vi "check chassis status.vi"(8 "error in (no error)":errorcluster {"code" format="%.0x"}, 11 "resource name":string="PXI11::0::0::INSTR" caption="resource string") -> (0 "error out":errorcluster {"code" format="%.0x"}, 3 "Status OK":bool)   [LabVIEW 2023]
uses:
  Program Files (x86)/Keysight/MPxiChassis/LabVIEW Driver/20xx/Keysight MPxiChassis/Keysight MPxiChassis.lvlib
panel:
  out "AlarmOccurred":bool caption="ClockAlarmOccurred"
  out "Clock source":i32=2
  # "0 10MHz from chassis\n1 10MHz clock from external\n2 10MHz from timing module\n3 10MHz clock from high performance reference\n4 2.4GHz clock from high performance reference"
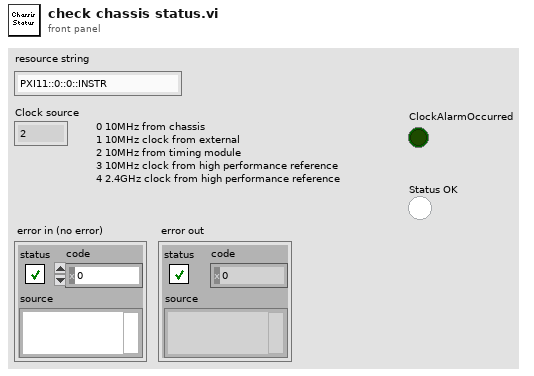
[diagram p1: front panel]
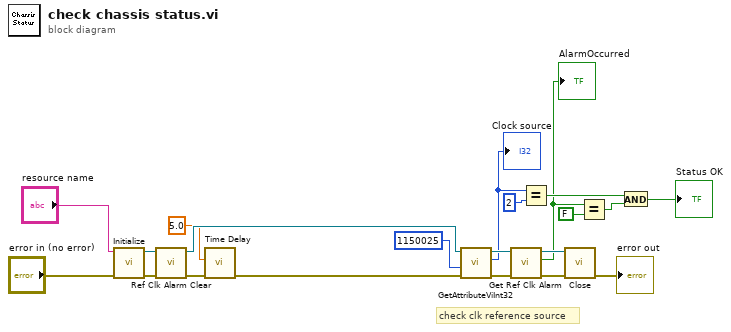
[diagram p0: block diagram]
diagram:
  # "check clk reference source"
  n1 = call "Initialize.vi"("error in (no error)"="error in (no error)", "resource name"="resource name") -> ("error out"=w4:errorcluster, "instrument handle out"=w6:refnum<k15>)  [unwired: 8 in]
  n2 = call "Ref Clk Alarm Clear.vi"("error in (no error)"=w4, "instrument handle"=w6) -> ("error out"=w2:errorcluster, "instrument handle out"=w5:refnum<k15>)  [unwired: 8 in]
  n3 = call "Time Delay"("error in (no error)"=w2, "Delay Time (s)"=5.0) -> ("error out"=w1:errorcluster)  [unwired: 9 in]
  n4 = call "GetAttributeViInt32.vi"("error in (no error)"=w1, "Attribute ID"=u32 1150025, "instrument handle"=w5) -> ("error out"=w17:errorcluster, "AttributeValue"=w13:i32, "instrument handle out"=w18:refnum<k15>)  [unwired: 6 in]
  "Clock source" <- w13
  n5 = call "Get Ref Clk Alarm.vi"("error in (no error)"=w17, "instrument handle"=w18) -> ("error out"=w15:errorcluster, "AlarmOccurred"=w10:bool, "instrument handle out"=w16:refnum<k15>)  [unwired: 7 in]
  "AlarmOccurred" <- w10
  n6 = Equal?(x=w13, y=2) -> (x = y?=w11:bool)
  n7 = call "Close.vi"("error in (no error)"=w15, "instrument handle"=w16) -> ("error out"=→"error out":errorcluster)  [unwired: 9 in]
  n8 = Equal?(x=w10, y=FALSE) -> (x = y?=w8:bool)
  n9 = And(x=w11, y=w8) -> (x .and. y?=→"Status OK":bool)
